vi "read map.vi"(1 "select file":path) -> (0 "Map Data":T1)   [LabVIEW 2009]
uses:
  <vilib>/regexp/Match Regular Expression.xnode
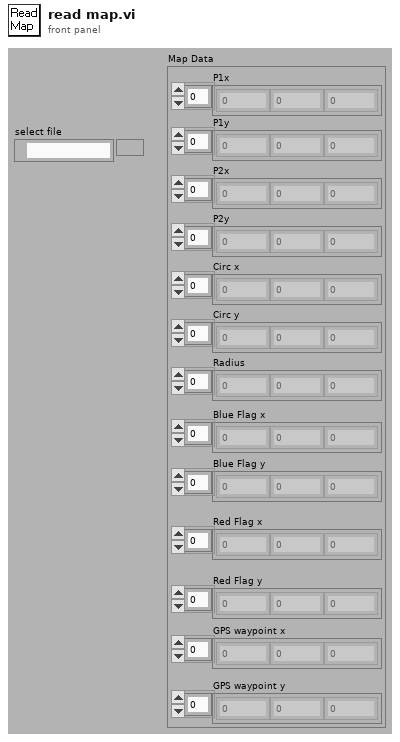
[diagram p1: front panel]
types:
  T1 = cluster{"P1x":dbl[], "P1y":dbl[], "P2x":dbl[], "P2y":dbl[], "Circ x":dbl[], "Circ y":dbl[], "Radius":dbl[], "Blue Flag x":dbl[], "Blue Flag y":dbl[], "Red Flag x":dbl[], "Red Flag y":dbl[], "GPS waypoint x":dbl[], "GPS waypoint y":dbl[]}
  T2 = enum16{"open", "replace", "create", "open or create", "replace or create", "replace or create with confirmation"}
  T3 = cluster{dbl[], dbl[], dbl[], dbl[], dbl[], dbl[], dbl[], dbl[], dbl[], dbl[], dbl[], dbl[], dbl[]}
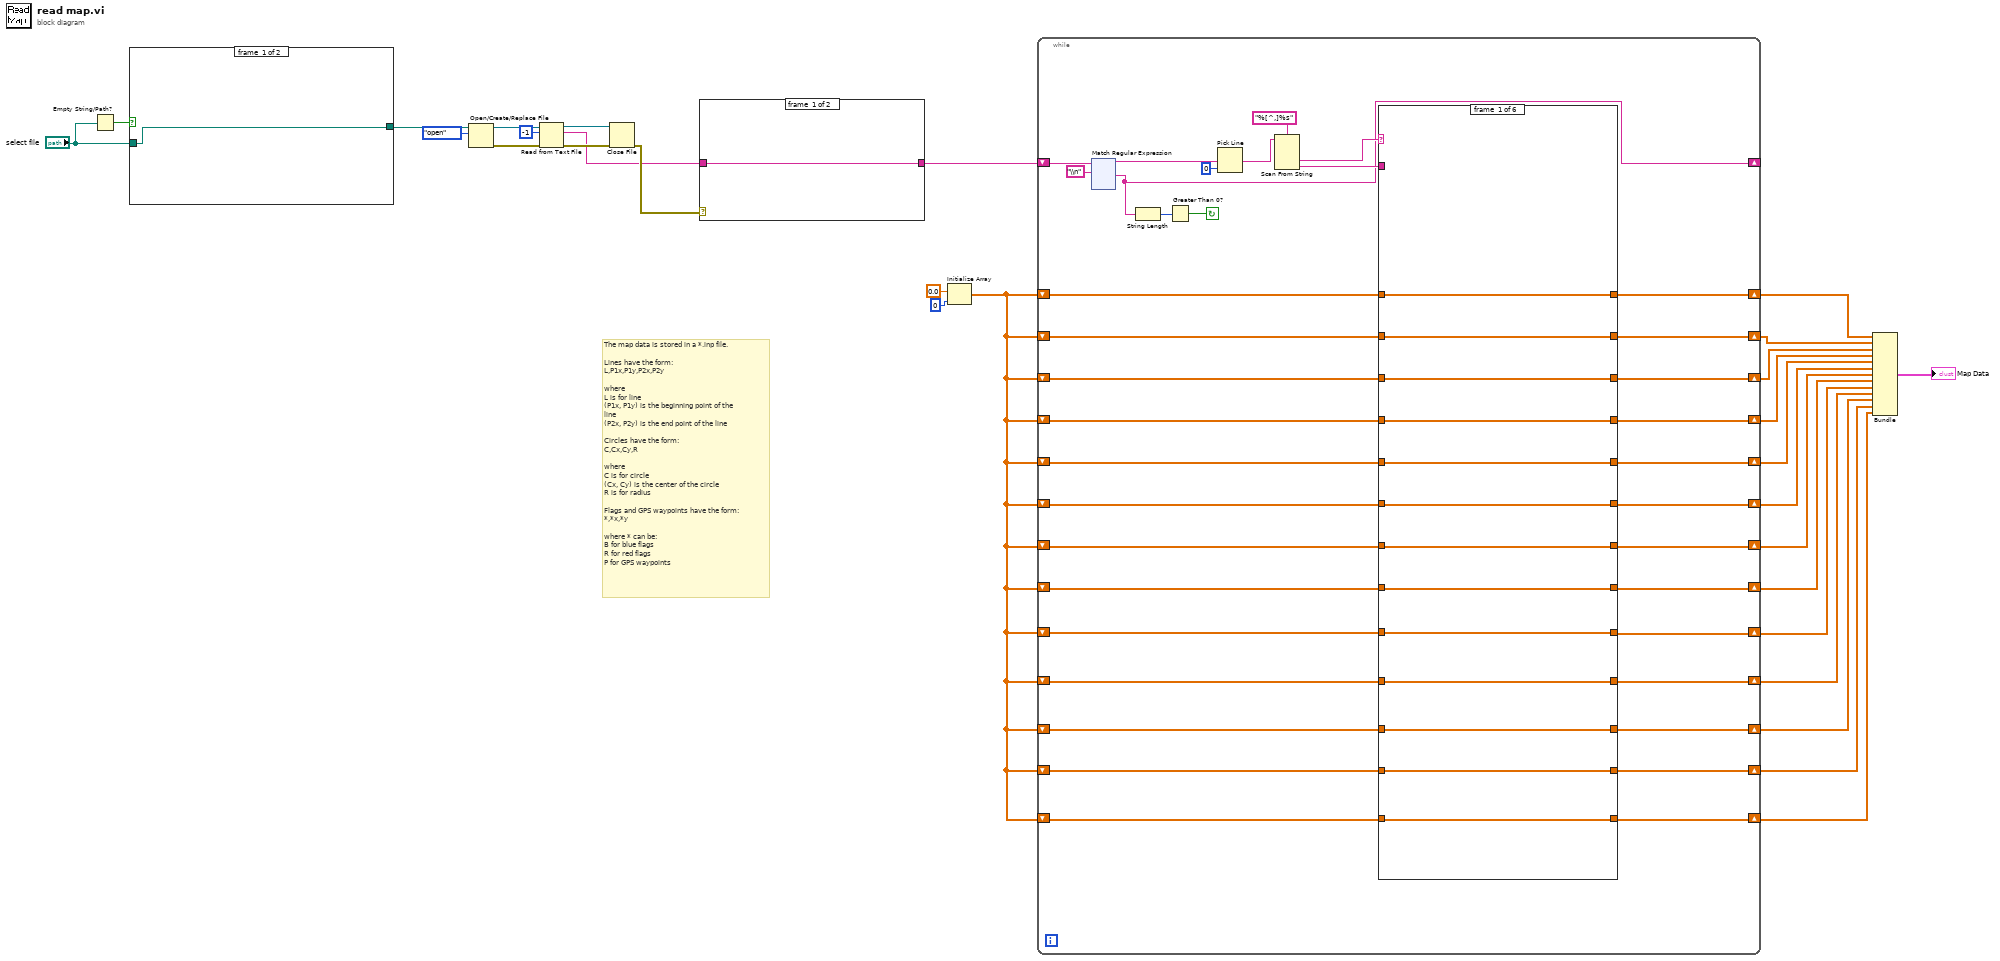
[diagram p0: block diagram]
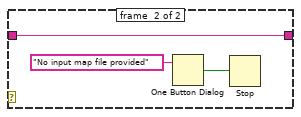
[diagram p2: hidden frame]
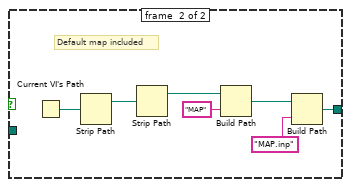
[diagram p3: hidden frame]
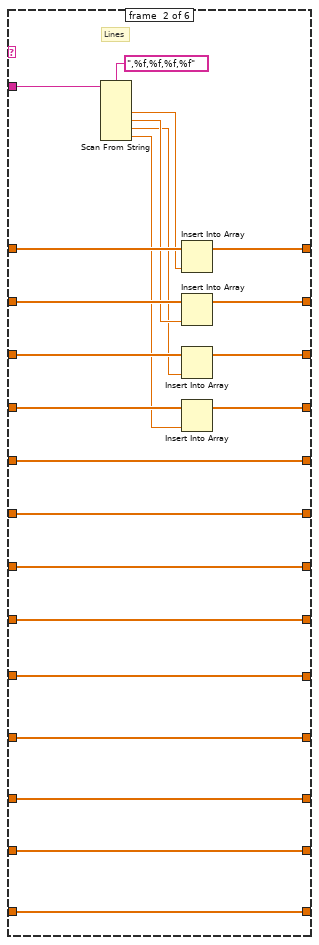
[diagram p4: hidden frame]
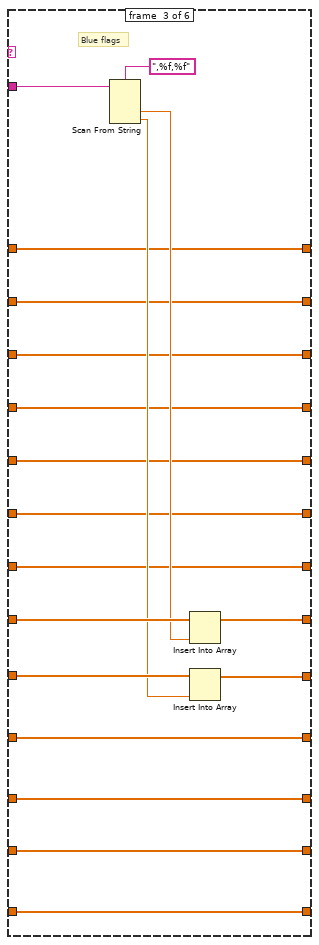
[diagram p5: hidden frame]
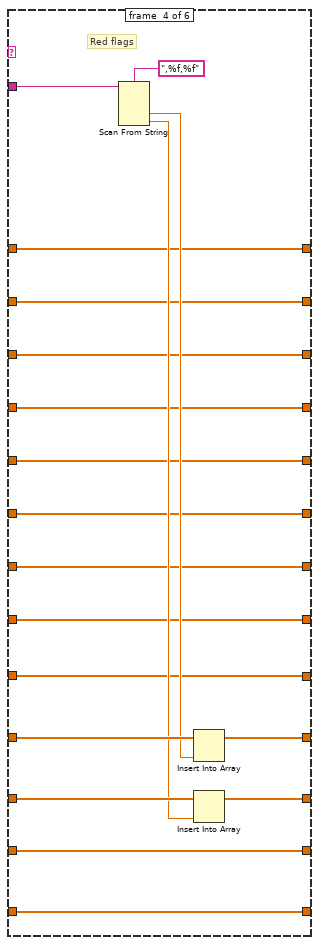
[diagram p6: hidden frame]
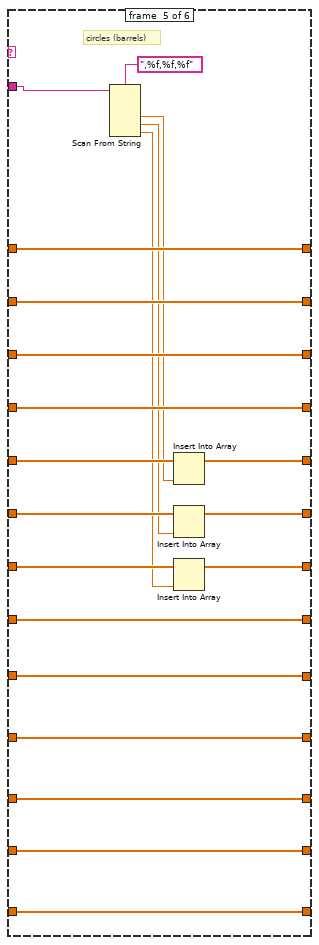
[diagram p7: hidden frame]
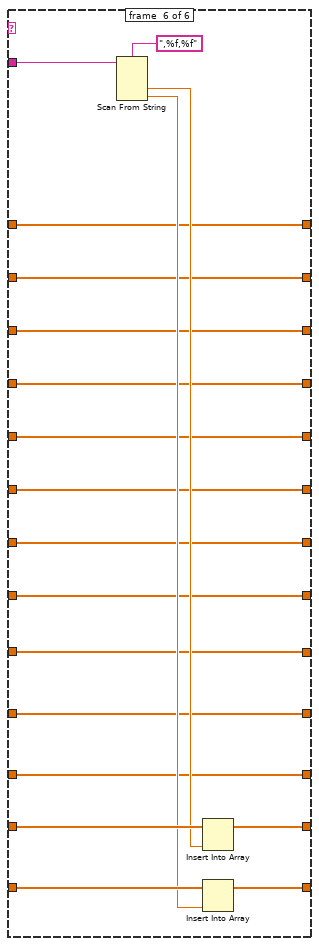
[diagram p8: hidden frame]
diagram:
  # "The map data is stored in a *.inp file.\n\nLines have the form:\nL,P1x,P1y,P2x,P2y\n\nwhere\nL is for line\n(P1x, P1y) is the beginning point of the line\n(P2x, P2y) is the end point of the line\n\nCircles have the form:\nC,Cx,Cy,R\n\nwhere\nC is for circle\n(Cx, Cy) is the center of the circle\nR is for radius\n\nFlags and GPS waypoints have the form:\n*,*x,*y\n\nwhere * can be:\nB for blue flags\nR for red flags\nP for GPS waypoints"
  n1 = Empty String/Path?(string/path="select file") -> (empty?=w13:bool)
  n2 = case shown="False" w13 {
    tunnel: [w30 w31] -> w14
    tunnel: "select file" -> [w30 _]
    frame #0 {
    }
    frame #1 {
      # "Default map included"
      n3 = Current VI's Path() -> (path=w37:path)
      n4 = Strip Path(path=w37) -> (stripped path=w34:path)  [unwired: 1 out]
      n5 = Strip Path(path=w34) -> (stripped path=w33:path)  [unwired: 1 out]
      n6 = Build Path(base path=w33, name or relative path="MAP") -> (appended path=w32:path)
      n7 = Build Path(base path=w32, name or relative path="MAP.inp") -> (appended path=w31:path)
    }
  }
  n8 = Open/Create/Replace File(file path (use dialog)=w14, operation (0:open)=T2."open") -> (refnum out=w28:refnum<file>, error out=w27:errorcluster)  [unwired: 4 in, 1 out]
  n9 = Read from Text File(file (use dialog)=w28, count=-1, error in=w27) -> (refnum out=w25:refnum<file>, text=w10:string, error out=w24:errorcluster)  [unwired: 1 in, 1 out]
  n10 = Close File(refnum=w25, error in=w24) -> (error out=w11:errorcluster)  [unwired: 1 out]
  n11 = case shown="No Error" w11 {
    tunnel: w10 -> [w38 w39]
    tunnel: [w38 w39] -> w9
    frame #0 {
    }
    frame #1 {
      n12 = One Button Dialog(message="No input map file provided") -> (true=w40:bool)  [unwired: 1 in]
      n13 = Stop(stop? (T)=w40) -> ()
    }
  }
  n14 = Initialize Array(0.0 ("element"), 0 ("dimension size")) -> (w4:dbl[])
  n15 = while {
    shift-right: [w66] -> _
    shift-left: w9 -> [w76]
    shift-right: [w67] -> w21
    shift-left: w4 -> [w68]
    shift-right: [w62] -> w20
    shift-left: w4 -> [w65]
    shift-right: [w61] -> w19
    shift-left: w4 -> [w64]
    shift-right: [w60] -> w18
    shift-left: w4 -> [w63]
    shift-right: [w56] -> w17
    shift-left: w4 -> [w59]
    shift-right: [w55] -> w16
    shift-left: w4 -> [w58]
    shift-right: [w54] -> w15
    shift-left: w4 -> [w57]
    shift-right: [w53] -> w8
    shift-left: w4 -> [w52]
    shift-right: [w50] -> w7
    shift-left: w4 -> [w51]
    shift-right: [w47] -> w6
    shift-left: w4 -> [w49]
    shift-right: [w46] -> w5
    shift-left: w4 -> [w48]
    shift-right: [w44] -> w3
    shift-left: w4 -> [w45]
    shift-right: [w42] -> w2
    shift-left: w4 -> [w43]
    stop <- w75 continue-if-true
    n16 = xnode "Match Regular Expression"("input string"=w76, "regular expression"="\\n") -> ("before match"=w69:string, "after match"=w66:string)  [unwired: 4 in, 3 out]
    n17 = String Length(string=w66) -> (length=w77:i32)
    n18 = Greater Than 0?(x=w77) -> (x > 0?=w75:bool)
    n19 = Pick Line(multi-line string=w69, line index=0) -> (output string=w71:string)  [unwired: 1 in]
    n20 = Scan From String(format string="%[^,]%s", input string=w71) -> (output 1=w74:string, output 2=w73:string)  [unwired: 4 in, 3 out]
    n21 = case shown="\"R\"" w74 {
      tunnel: w73 -> [_ w113 w132 w151 w172 w191]
      tunnel: w68 -> [w91 w112 w125 w144 w171 w174]
      tunnel: [w91 w111 w125 w144 w171 w174] -> w67
      tunnel: w65 -> [w90 w110 w124 w143 w170 w175]
      tunnel: w64 -> [w89 w109 w123 w142 w169 w176]
      tunnel: w63 -> [w88 w108 w122 w141 w168 w177]
      tunnel: [w90 w106 w124 w143 w170 w175] -> w62
      tunnel: [w89 w105 w123 w142 w169 w176] -> w61
      tunnel: [w88 w104 w122 w141 w168 w177] -> w60
      tunnel: w59 -> [w87 w100 w121 w140 w167 w178]
      tunnel: w58 -> [w86 w99 w120 w139 w166 w179]
      tunnel: w57 -> [w85 w98 w119 w138 w165 w180]
      tunnel: [w87 w100 w121 w140 w161 w178] -> w56
      tunnel: [w86 w99 w120 w139 w160 w179] -> w55
      tunnel: [w85 w98 w119 w138 w159 w180] -> w54
      tunnel: [w84 w97 w129 w137 w158 w181] -> w53
      tunnel: w52 -> [w84 w97 w131 w137 w158 w181]
      tunnel: w51 -> [w83 w96 w128 w136 w157 w182]
      tunnel: [w83 w96 w127 w136 w157 w182] -> w50
      tunnel: w49 -> [w82 w95 w118 w150 w156 w183]
      tunnel: w48 -> [w81 w94 w117 w149 w155 w184]
      tunnel: [w81 w94 w117 w148 w155 w184] -> w46
      tunnel: [w82 w95 w118 w147 w156 w183] -> w47
      tunnel: [w80 w93 w116 w135 w154 w188] -> w44
      tunnel: w45 -> [w80 w93 w116 w135 w154 w190]
      tunnel: [w79 w92 w115 w134 w153 w187] -> w42
      tunnel: w43 -> [w79 w92 w115 w134 w153 w189]
      frame #0 {
      }
      frame #1 {
        # "Lines"
        n22 = Scan From String(format string=",%f,%f,%f,%f", input string=w113) -> (output 1=w107:dbl, output 2=w103:dbl, output 3=w102:dbl, output 4=w101:dbl)  [unwired: 6 in, 3 out]
        n23 = Insert Into Array(array=w112, new element=w107) -> (w111:dbl[])  [unwired: 1 in]
        n24 = Insert Into Array(array=w110, new element=w103) -> (w106:dbl[])  [unwired: 1 in]
        n25 = Insert Into Array(array=w109, new element=w102) -> (w105:dbl[])  [unwired: 1 in]
        n26 = Insert Into Array(array=w108, new element=w101) -> (w104:dbl[])  [unwired: 1 in]
      }
      frame #2 {
        # "Blue flags"
        n27 = Scan From String(format string=",%f,%f", input string=w132) -> (output 1=w130:dbl, output 2=w126:dbl)  [unwired: 4 in, 3 out]
        n28 = Insert Into Array(array=w131, new element=w130) -> (w129:dbl[])  [unwired: 1 in]
        n29 = Insert Into Array(array=w128, new element=w126) -> (w127:dbl[])  [unwired: 1 in]
      }
      frame #3 {
        # "Red flags"
        n30 = Scan From String(format string=",%f,%f", input string=w151) -> (output 1=w146:dbl, output 2=w145:dbl)  [unwired: 4 in, 3 out]
        n31 = Insert Into Array(array=w150, new element=w146) -> (w147:dbl[])  [unwired: 1 in]
        n32 = Insert Into Array(array=w149, new element=w145) -> (w148:dbl[])  [unwired: 1 in]
      }
      frame #4 {
        # "circles (barrels)"
        n33 = Scan From String(format string=",%f,%f,%f", input string=w172) -> (output 1=w163:dbl, output 2=w162:dbl, output 3=w164:dbl)  [unwired: 5 in, 3 out]
        n34 = Insert Into Array(array=w167, new element=w163) -> (w161:dbl[])  [unwired: 1 in]
        n35 = Insert Into Array(array=w166, new element=w162) -> (w160:dbl[])  [unwired: 1 in]
        n36 = Insert Into Array(array=w165, new element=w164) -> (w159:dbl[])  [unwired: 1 in]
      }
      frame #5 {
        n37 = Scan From String(format string=",%f,%f", input string=w191) -> (output 1=w186:dbl, output 2=w185:dbl)  [unwired: 4 in, 3 out]
        n38 = Insert Into Array(array=w190, new element=w186) -> (w188:dbl[])  [unwired: 1 in]
        n39 = Insert Into Array(array=w189, new element=w185) -> (w187:dbl[])  [unwired: 1 in]
      }
    }
  }
  n40 = Bundle(w21, w20, w19, w18, w17, w16, w15, w8, w7, w6, w5, w3, w2) -> (→"Map Data":T3)  [unwired: 1 in]
